vi "To and From CSV Test.vi"() -> (0 "error out":errorcluster, 1 "Pass":bool, 2 "Lines Equal":bool, 3 "Class Equal":bool)   [LabVIEW 2015, in "PID Module tests.lvlib"]
uses:
  PID Module tests.lvlib
  <vilib>/NI/Module Execution Interface/Engine Configuration/engine configuration.lvclass
  editor node/PID Module editor node.lvclass
  module/configuration/PID Module configuration.lvclass
  module/configuration/PID Module configuration.lvclass/PID Module configuration.ctl
  <vilib>/NI/Configuration Framework/serializable configuration/NISE_CEF_serializable configuration.lvclass/NISE_CEF_serializable configuration.ctl
  <vilib>/Utility/LVClass/Get LV Class Name.vi
  <vilib>/NI/Configuration Framework/error generator/NISE_error generator.vi
  <vilib>/NI/Tag Bus Module Framework/channel/TBM channel.lvclass
  <vilib>/NI/Configuration Framework/serializable configuration/NISE_CEF_serializable configuration.lvclass
panel:
  out "x = y?":T1(array[cluster])
  out "Write Tags 2":string[](array[string])
  out "Write Tags 1":string[](array[string])
  out "Read Tags 1":string[](array[string])
  out "Read Tags 2":string[](array[string])
  out "To String Array 2":string[][](array[string])
  out "To String Array":string[][](array[string])
  out "Channels `":string[](array[string])
  out "Channels 2":string[](array[string])
  out "Write Channels":bool
  out "Read Channels":bool
  # "Lines"
  # "Channels"
  # "Tags"
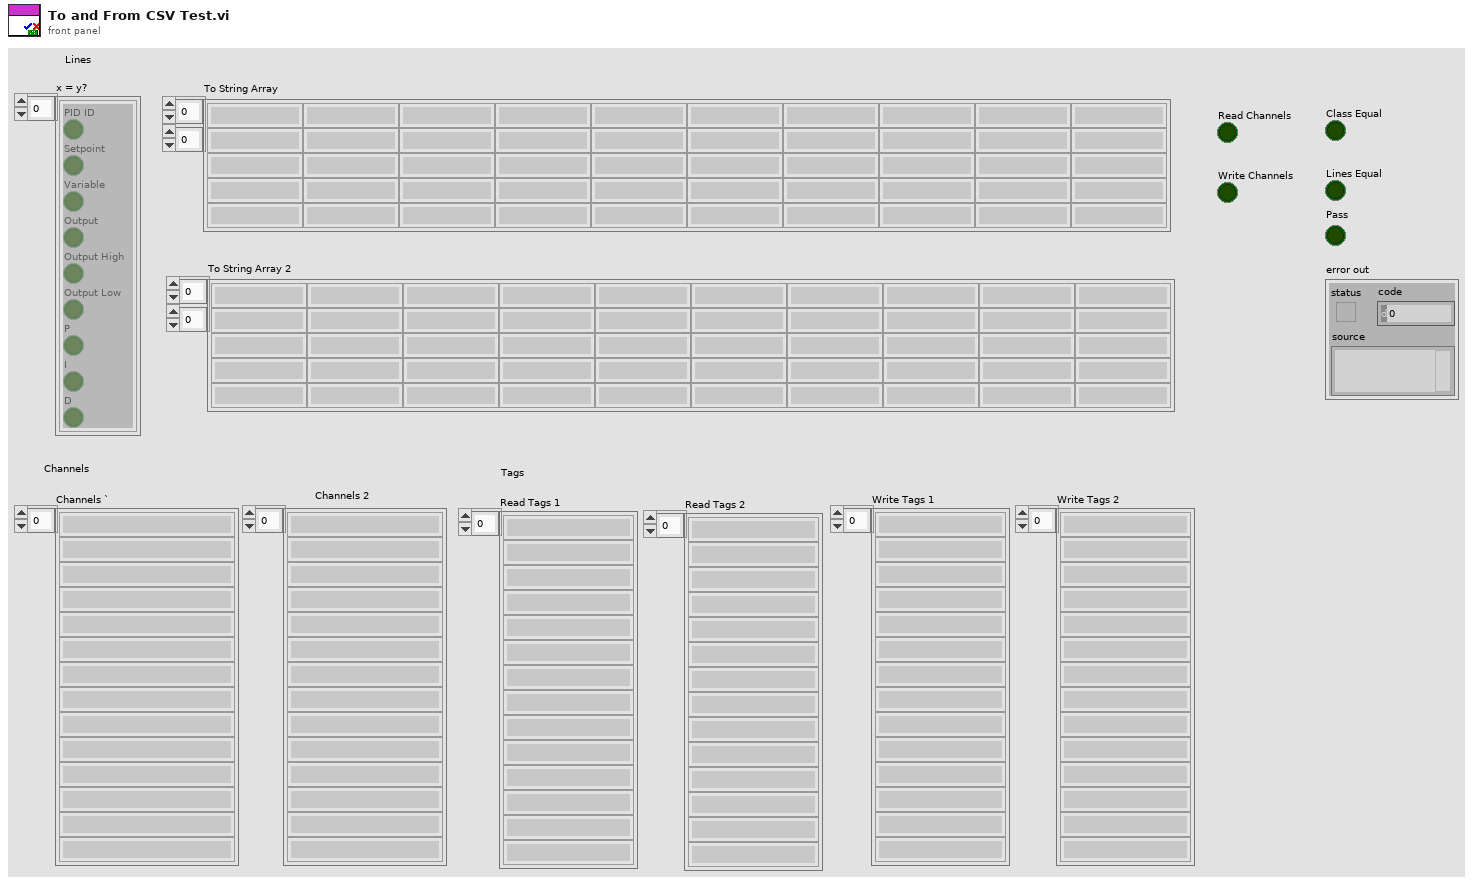
[diagram p1: front panel]
types:
  T1 = cluster{"PID ID":bool, "Setpoint":bool, "Variable":bool, "Output":bool, "Output High":bool, "Output Low":bool, "P":bool, "I":bool, "D":bool}[]
  T2 = typedef "PID Module configuration.lvclass/Line.ctl" = cluster{"PID ID":string, "Setpoint":refnum<class "TBM channel.lvclass">, "Variable":refnum<class "TBM channel.lvclass">, "Output":refnum<class "TBM channel.lvclass">, "Output High":refnum<class "TBM channel.lvclass">, "Output Low":refnum<class "TBM channel.lvclass">, "P":refnum<class "TBM channel.lvclass">, "I":refnum<class "TBM channel.lvclass">, "D":refnum<class "TBM channel.lvclass">}
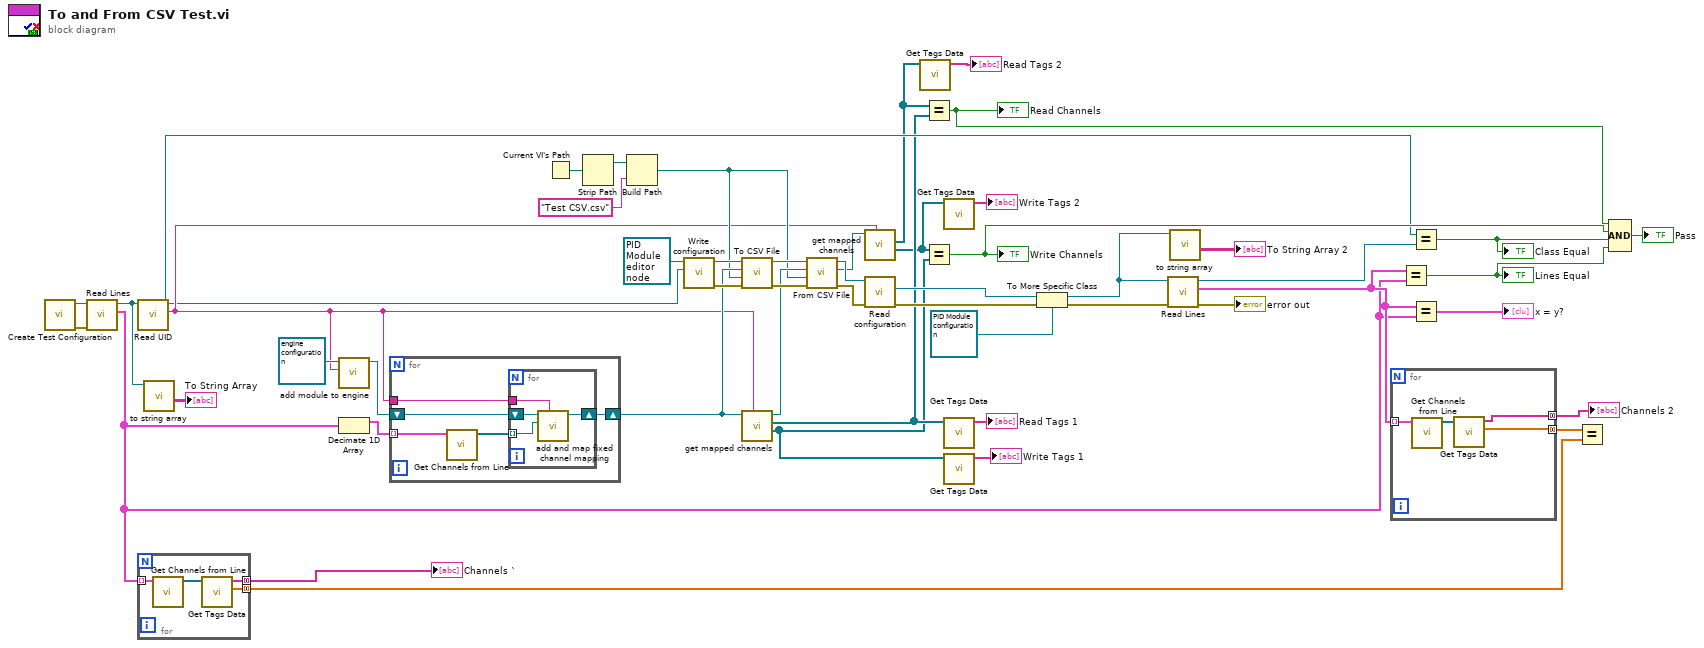
[diagram p0: block diagram]
diagram:
  n1 = call "Create Test Configuration.vi"() -> ("error out"=w50:errorcluster, "Module Configuration"=w51:refnum<class "PID Module configuration.lvclass">)  [unwired: 6 in, 4 out]
  n2 = call "Read Lines.vi"("error in (no error)"=w50, "PID Module configuration in"=w51) -> ("Lines"=w10:T2[], "PID Module configuration out"=w15:refnum<class "PID Module configuration.lvclass">)  [unwired: 7 in, 1 out]
  n3 = call <vilib>:"Read UID.vi"("configuration in"=w15) -> ("instance id"=w24:string, "configuration out"=w21:refnum<class "PID Module configuration.lvclass">)  [unwired: 8 in, 1 out]
  n4 = for {
    tunnel: w10 -> [w55] mode=indexing
    tunnel: [w53] -> w19 mode=concatenating
    tunnel: [w52] -> w17 mode=concatenating
    n5 = call "Get Channels from Line.vi"("Line"=w55) -> ("Channels"=w54:refnum<class "TBM channel.lvclass">[])  [unwired: 10 in]
    n6 = call "Get Tags Data.vi"("Channels"=w54) -> ("Array"=w52:dbl[], "Array 2"=w53:string[])  [unwired: 9 in]
  }
  "Channels `" <- w19
  n7 = call-dynamic "to string array.vi"("PID Module configuration in"=w15) -> ("Array"=→"To String Array":string[][])  [unwired: 7 in, 3 out]
  n8 = call-dynamic "add module to engine.vi"("module ID"=w24, "engine configuration in"=refnum<class "engine configuration.lvclass"> refnum ("engine configuration")) -> ("engine configuration out"=w43:refnum<class "engine configuration.lvclass">)  [unwired: 8 in, 1 out]
  n9 = Decimate 1D Array(w10) -> (w12:T2[])  [unwired: 1 out]
  n10 = for {
    tunnel: w12 -> [w57] mode=indexing
    tunnel: w24 -> [w60]
    shift-right: [w59] -> w35
    shift-left: w43 -> [w58]
    n11 = call "Get Channels from Line.vi"("Line"=w57) -> ("Channels"=w56:refnum<class "TBM channel.lvclass">[])  [unwired: 10 in]
    n12 = for {
      tunnel: w60 -> [w64]
      shift-right: [w63] -> w59
      shift-left: w58 -> [w62]
      tunnel: w56 -> [w61] mode=indexing
      n13 = call <vilib>:"add and map fixed channel mapping.vi"("module instance"=w64, "fixed channel"=w61, "engine configuration in"=w62) -> ("engine configuration out"=w63:refnum<class "engine configuration.lvclass">)  [unwired: 7 in, 1 out]
    }
  }
  n14 = Current VI's Path() -> (path=w32:path)
  n15 = Strip Path(path=w32) -> (stripped path=w31:path)  [unwired: 1 out]
  n16 = Build Path(base path=w31, name or relative path="Test CSV.csv") -> (appended path=w30:path)
  n17 = call-dynamic "Write configuration.vi"("configuration"=w21, "PID Module editor node in"=refnum<class "PID Module editor node.lvclass"> refnum ("tag bus configurable plugin editor node")) -> ("error out"=w37:errorcluster, "PID Module editor node out"=w42:refnum<class "PID Module editor node.lvclass">)  [unwired: 8 in]
  n18 = call-dynamic "To CSV File.vi"("error in (no error)"=w37, "Path"=w30, "engine configuration"=w35, "PID Module editor node in"=w42) -> ("error out"=w38:errorcluster, "PID Module editor node out"=w40:refnum<class "PID Module editor node.lvclass">)  [unwired: 6 in]
  n19 = call-dynamic "get mapped channels.vi"("owner"=w24, "engine configuration in"=w35) -> ("write channels"=w6:refnum<class "TBM channel.lvclass">[], "read channels"=w8:refnum<class "TBM channel.lvclass">[], "engine configuration out"=w34:refnum<class "engine configuration.lvclass">)  [unwired: 5 in, 2 out]
  n20 = call-dynamic "From CSV File.vi"("error in (no error)"=w38, "Path"=w30, "engine in"=w34, "PID Module editor node in"=w40) -> ("error out"=w39:errorcluster, "engine out"=w29:refnum<class "engine configuration.lvclass">, "PID Module editor node out"=w41:refnum<class "PID Module editor node.lvclass">)  [unwired: 4 in, 1 out]
  n21 = call-dynamic "get mapped channels.vi"("owner"=w24, "engine configuration in"=w29) -> ("write channels"=w2:refnum<class "TBM channel.lvclass">[], "read channels"=w4:refnum<class "TBM channel.lvclass">[])  [unwired: 5 in, 3 out]
  n22 = call-dynamic "Read configuration.vi"("error in"=w39, "PID Module editor node in"=w41) -> ("error out"=w26:errorcluster, "configuration"=w27:refnum<class "NISE_CEF_serializable configuration.lvclass">)  [unwired: 7 in, 1 out]
  n23 = call "Get Tags Data.vi"("Channels"=w4) -> ("Array 2"=→"Read Tags 2":string[])  [unwired: 9 in, 1 out]
  n24 = Equal?(x=w4, y=w8) -> (x = y?=w45:bool)
  "Read Channels" <- w45
  n25 = Equal?(x=w2, y=w6) -> (x = y?=w44:bool)
  "Write Channels" <- w44
  n26 = call "Get Tags Data.vi"("Channels"=w2) -> ("Array 2"=→"Write Tags 2":string[])  [unwired: 9 in, 1 out]
  n27 = call "Get Tags Data.vi"("Channels"=w8) -> ("Array 2"=→"Read Tags 1":string[])  [unwired: 9 in, 1 out]
  n28 = call "Get Tags Data.vi"("Channels"=w6) -> ("Array 2"=→"Write Tags 1":string[])  [unwired: 9 in, 1 out]
  n29 = To More Specific Class(target class=refnum<class "PID Module configuration.lvclass"> refnum ("tag bus configurable plugin module configuration"), reference=w27, error in=w26) -> (specific class reference=w13:refnum<class "PID Module configuration.lvclass">, error out=w25:errorcluster)
  n30 = call "Read Lines.vi"("error in (no error)"=w25, "PID Module configuration in"=w13) -> ("error out"=→"error out":errorcluster, "Lines"=w11:T2[], "PID Module configuration out"=w49:refnum<class "PID Module configuration.lvclass">)  [unwired: 7 in]
  n31 = call-dynamic "to string array.vi"("PID Module configuration in"=w13) -> ("Array"=→"To String Array 2":string[][])  [unwired: 7 in, 3 out]
  n32 = for {
    tunnel: w11 -> [w68] mode=indexing
    tunnel: [w66] -> w20 mode=concatenating
    tunnel: [w65] -> w18 mode=concatenating
    n33 = call "Get Channels from Line.vi"("Line"=w68) -> ("Channels"=w67:refnum<class "TBM channel.lvclass">[])  [unwired: 10 in]
    n34 = call "Get Tags Data.vi"("Channels"=w67) -> ("Array"=w65:dbl[], "Array 2"=w66:string[])  [unwired: 9 in]
  }
  "Channels 2" <- w20
  n35 = Equal?(x=w11, y=w10) -> (x = y?=w22:bool)
  "Lines Equal" <- w22
  n36 = Equal?(x=w21, y=w49) -> (x = y?=w23:bool)
  "Class Equal" <- w23
  n37 = Equal?(x=w11, y=w10) -> (x = y?=→"x = y?":T1)
  n38 = Equal?(x=w18, y=w17) -> ()  [unwired: 1 out]
  n39 = Compound Arithmetic op=AND(w45, w44, w23, w22) -> (→"Pass":bool)
